vi "Mono (YJ 20190218).vi"() -> ()   [LabVIEW 2017]
uses:
  C:/Users/Admin/Desktop/S-EQE (YJ)/Mono vi (YJ)/Cornerstone.dll
  Cornerstone.dll
panel:
  in  "stop":bool
  out "Wavelength Range":dbl[](array[numeric])
  in  "Step size (nm)":sgl=5.0 min=1 step=0.1
  in  "End Wavelength (nm)":dbl=1000.0 min=250.0 max=1350.0 step=0.1
  in  "Start Wavelength (nm)":dbl=350.0 min=250.0 max=1200.0 step=0.1
  out "CmdLib (Mono)":refnum<k24>
  out "Mono status":bool
  out "Current Wavelength":dbl=999.986 min=350.0 max=1100.0 step=1.0 format="%#.1f"
  in  "Start Wavelength (nm)":dbl=350.0 min=250.0 max=1200.0 step=0.1
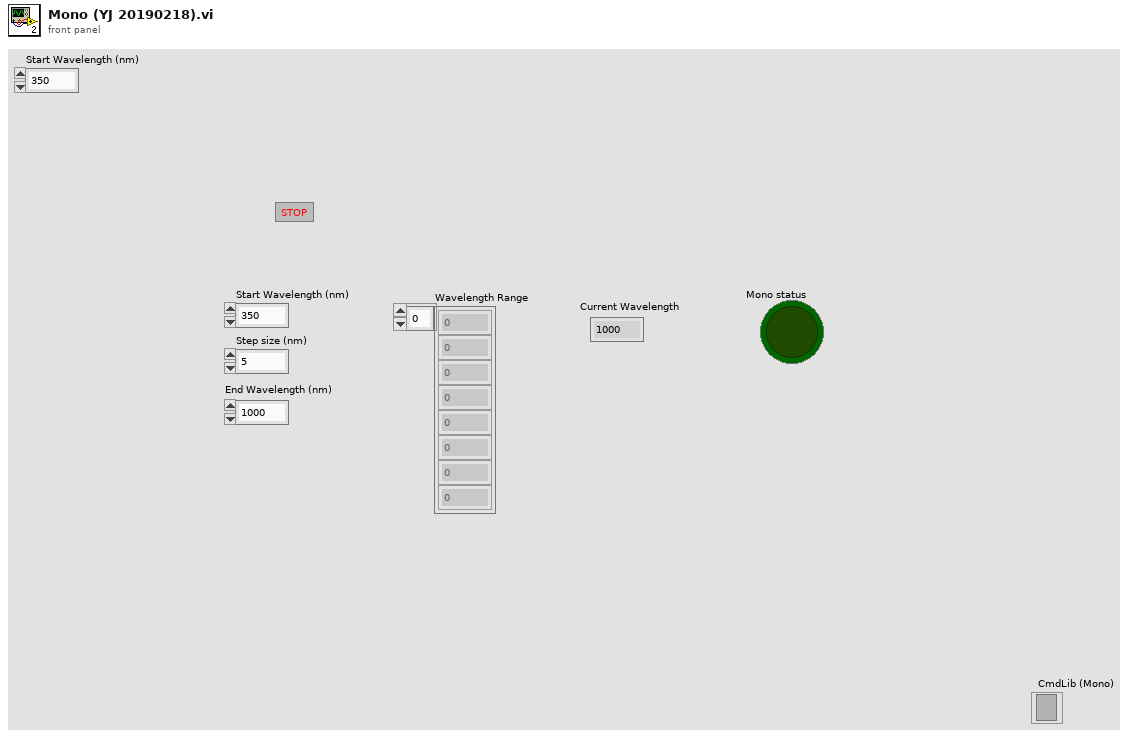
[diagram p1: front panel]
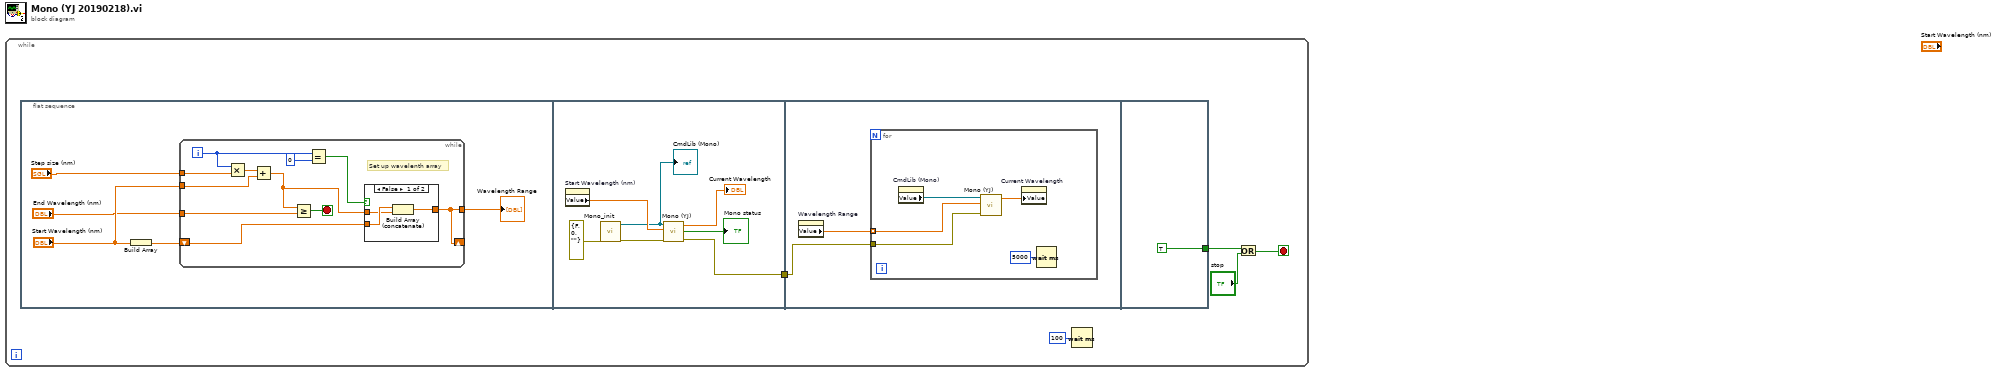
[diagram p0: block diagram]
diagram:
  n1 = while {
    stop <- w2 stop-if-true
    n2 = flat-sequence {
      tunnel: [w26] -> w5
      tunnel: w5 -> [w33]
      tunnel: [TRUE] -> w4
      frame #0 {
        n3 = Build Array "Build Array"("Start Wavelength (nm)") -> (w10:dbl[])
        n4 = while {
          shift-right: [w11] -> _
          shift-left: w10 -> [w13]
          tunnel: "Step size (nm)" -> [w20]
          tunnel: "End Wavelength (nm)" -> [w21]
          tunnel: "Start Wavelength (nm)" -> [w14]
          tunnel: [w11] -> w6
          i -> [w16]
          stop <- w18 stop-if-true
          # "Set up wavelenth array"
          n5 = Multiply(x=w16, y=w20) -> (x*y=w19:sgl)
          n6 = Add(x=w19, y=w14) -> (x+y=w12:dbl)
          n7 = Greater Or Equal?(x=w12, y=w21) -> (x >= y?=w18:bool)
          n8 = Equal?(x=w16, y=0) -> (x = y?=w15:bool)
          n9 = case shown="False" w15 {
            tunnel: w13 -> [w24 w25]
            tunnel: w12 -> [w23 _]
            tunnel: [w22 w25] -> w11
            frame False {
              n10 = Build Array (concatenate)(w24, w23) -> (w22:dbl[])
            }
            frame True {
            }
          }
        }
        "Wavelength Range" <- w6
      }
      frame #1 {
        n11 = property on="Start Wavelength (nm)" class="DigNum (strict)"() -> ("Value"=w32:dbl)  [unwired: 2 in, 2 out]
        n12 = call "Mono_init.vi"("error in (no error)"=errorcluster {"status"=FALSE, "code"=0, "source"=""}) -> ("error out"=w29:errorcluster, "CmdLib"=w28:refnum<k24>)  [unwired: 8 in, 1 out]
        "CmdLib (Mono)" <- w28
        n13 = call "Mono (YJ).vi"("error in (no error)"=w29, "Go to Wavelength"=w32, "CmdLib In"=w28) -> ("error out 2"=w26:errorcluster, "State of Mono_SetWavelength"=→"Mono status":bool, "Current Wavelength"=→"Current Wavelength":dbl)  [unwired: 1 in]
      }
      frame #2 {
        n14 = property on="Wavelength Range" class="Arr (strict)"() -> ("Value"=w34:dbl[])  [unwired: 2 in, 2 out]
        n15 = for {
          tunnel: w34 -> [w37] mode=indexing
          tunnel: w33 -> [w38]
          n16 = property on="CmdLib (Mono)" class="Ref (strict)"() -> ("Value"=w39:refnum<k24>)  [unwired: 2 in, 2 out]
          n17 = call "Mono (YJ).vi"("error in (no error)"=w38, "Go to Wavelength"=w37, "CmdLib In"=w39) -> ("Current Wavelength"=w35:dbl)  [unwired: 1 in, 2 out]
          n18 = property on="Current Wavelength" class="DigNum (strict)"("Value"=w35) -> ()  [unwired: 2 in, 2 out]
          n19 = Wait (ms)(milliseconds to wait=u32 5000) -> ()  [unwired: 1 out]
        }
      }
      frame #3 {
      }
    }
    n20 = Wait (ms)(milliseconds to wait=u32 100) -> ()  [unwired: 1 out]
    n21 = Or(x=w4, y="stop") -> (x .or. y?=w2:bool)
  }
